vi "Write Acceleration.vi"(8 "error in (no error)":errorcluster, 10 "Acceleration":dbl, 11 "Configure Acceleration Msg in":refnum<class "Configure Acceleration Msg.lvclass">) -> (0 "error out":errorcluster, 3 "Configure Acceleration Msg out":refnum<class "Configure Acceleration Msg.lvclass">)   [LabVIEW 2015, in "CS++Motor.lvlib" / "Configure Acceleration Msg.lvclass"]
uses:
  Configure Acceleration Msg.lvclass
  Configure Acceleration Msg.lvclass/Configure Acceleration Msg.ctl
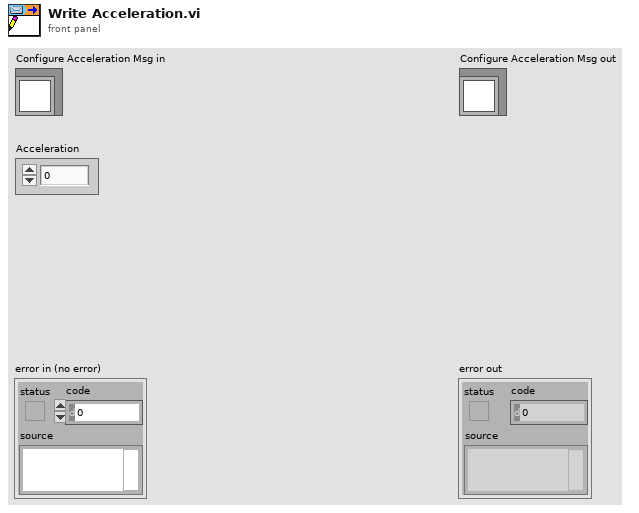
[diagram p1: front panel]
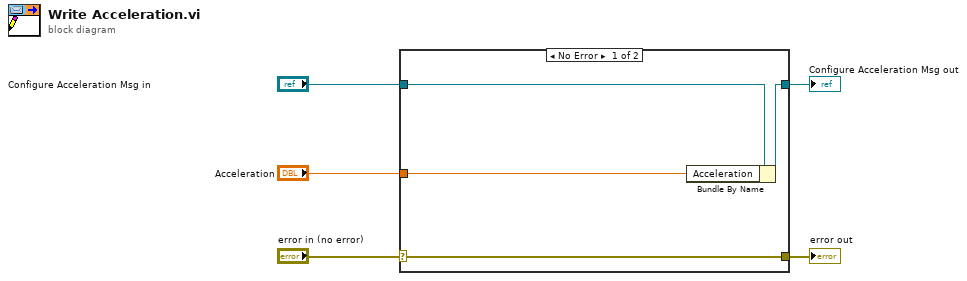
[diagram p0: block diagram]
diagram:
  n1 = case shown="No Error" "error in (no error)" {
    selector: "error in (no error)" -> [w9 w10]
    tunnel: [w9 w10] -> w4
    tunnel: [w7 w11] -> w2
    tunnel: "Configure Acceleration Msg in" -> [w8 w11]
    tunnel: "Acceleration" -> [w6 _]
    frame No Error {
      n2 = Bundle By Name(cluster=w8, "Acceleration"=w6) -> (w7:refnum<class "Configure Acceleration Msg.lvclass">)
    }
    frame Error {
    }
  }
  "error out" <- w4
  "Configure Acceleration Msg out" <- w2
